vi "RydbergExpControl_2014.8.27_beta.vi"() -> ()   [LabVIEW 2013]
uses:
  AndorCamera/camera_controls.ctl
  <userlib>/atmcd32d.llb/AcquisitionMode_mode typedef.ctl
  <userlib>/atmcd32d.llb/TriggerMode_mode typedef.ctl
  6704/6704_static_voltages_control.ctl
  rydberg_state_machine_states.ctl
panel:
  out "Atom Closeup":dbl[][](graph)
  out "Atoms - BG":dbl[][](graph)
  out "error out":errorcluster
  out "error constant":errorcluster
  out "Array":dbl[](array[numeric])
  out "Background Image":i16[][](graph)
  out "Atom Image":i16[][](graph)
  in  "Tab Control":T1(tab)
  in  "Trigger Snap Mode":bool
  out "Camera Ready":bool
  in  "Scan Name":string
  in  "Raw_Data Folder":path
  out "Exp Running":bool
  in  "PB Instruction Time To Change":i32
  in  "Static Channel To Change":i32
  in  "Step Size":dbl min=1e-06
  in  "Final Value":dbl
  in  "Initial Value":dbl
  out "You Are Changing:":string
  in  "Shutdown Experiment":bool
  in  "Start Experiment":bool
  in  "Instructions":T2(array[cluster])=[{"Instruct Data"=0, "Op Code"=0, "Flags"=[TRUE, FALSE, FALSE, FALSE, FALSE, FALSE, FALSE, FALSE, FALSE, FALSE, FALSE, FALSE, FALSE, FALSE, FALSE, FALSE, FALSE, FALSE, FALSE, FALSE, FALSE, FALSE, FALSE, FALSE], "Comments"="", "Time (s)"=0.1}, {"Instruct Data"=0, "Op Code"=0, "Flags"=[FALSE, FALSE, FALSE, FALSE, FALSE, FALSE, FALSE, FALSE, FALSE, FALSE, FALSE, FALSE, FALSE, FALSE, FALSE, FALSE, FALSE, FALSE, FALSE, FALSE, FALSE, FALSE, FALSE, FALSE], "Comments"="", "Time (s)"=0.1}, {"Instruct Data"=0, "Op Code"=0, "Flags"=[TRUE, FALSE, FALSE, FALSE, FALSE, FALSE, FALSE, FALSE, FALSE, FALSE, FALSE, FALSE, FALSE, FALSE, FALSE, FALSE, FALSE, FALSE, FALSE, FALSE, FALSE, FALSE, FALSE, FALSE], "Comments"="", "Time (s)"=0.1}, {"Instruct Data"=0, "Op Code"=6, "Flags"=[FALSE, FALSE, FALSE, FALSE, FALSE, FALSE, FALSE, FALSE, FALSE, FALSE, FALSE, FALSE, FALSE, FALSE, FALSE, FALSE, FALSE, FALSE, FALSE, FALSE, FALSE, FALSE, FALSE, FALSE], "Comments"="", "Time (s)"=0.1}] {"Time (s)" format="%.3p"; "Op Code" items=["Continue", "Stop", "Loop", "End Loop", "JSR", "RTS", "Branch", "Long Delay", "Wait"]}
  in  "What To Change":enum16{"PulseBlaster", "Static Voltage"}(ring)=enum."Static Voltage"
  out "Scan Progress":dbl(slide) caption="Slide" scale=0.0..100.0
  out "Camera Information":T3 {"VS Speed (us)" format="%.2f"}
  in  "Acquisition Parameters":T4={"Acquisition Mode"=enum."Kinetics", "Trigger Mode"=enum."External", "Frame \nTransfer"=FALSE, "Exposure Time (s)"=0.0001, "Accumulation Cycle Time (s)"=0.0, "# Accumulations"=1, "# Kinetics"=2, "Kinetic Cycle Time (s)"=0.0, "Horizontal Bin Size"=1, "Vertical Bin Size"=1} {"Vertical Bin Size" min=1; "Horizontal Bin Size" min=1; "Kinetic Cycle Time (s)" format="%.2f"; "# Kinetics" min=1; "# Accumulations" min=1; "Accumulation Cycle Time (s)" format="%.2f"; "Exposure Time (s)" format="%.2e"}
  out "Calcualted Times":T7 {"Kinetic" format="%.4f"; "Accumulate" format="%.4f"; "Exposure" format="%.4f"}
  in  "Red MOT 87 Inputs":T8={"Active Device"="6733_Red_87", "Active Channels"=[TRUE, FALSE, FALSE, FALSE, FALSE, FALSE, FALSE, FALSE], "Waveform Parameters"=[[{"Functional Form"=enum."Polynomial", "Start Voltage"=0.0, "End Voltage"=0.0, "Time"=0.0, "Degree"=1, "Sample Rate"=0.0}, {"Functional Form"=enum."Exponential", "Start Voltage"=0.0, "End Voltage"=0.0, "Time"=0.0, "Degree"=1, "Sample Rate"=0.0}, {"Functional Form"=enum."Exponential", "Start Voltage"=0.0, "End Voltage"=0.0, "Time"=0.0, "Degree"=1, "Sample Rate"=0.0}, {"Functional Form"=enum."Exponential", "Start Voltage"=0.0, "End Voltage"=0.0, "Time"=0.0, "Degree"=1, "Sample Rate"=0.0}, {"Functional Form"=enum."Exponential", "Start Voltage"=0.0, "End Voltage"=0.0, "Time"=0.0, "Degree"=1, "Sample Rate"=0.0}, {"Functional Form"=enum."Exponential", "Start Voltage"=0.0, "End Voltage"=0.0, "Time"=0.0, "Degree"=1, "Sample Rate"=0.0}], [{"Functional Form"=enum."Exponential", "Start Voltage"=0.0, "End Voltage"=0.0, "Time"=0.0, "Degree"=1, "Sample Rate"=0.0}, {"Functional Form"=enum."Exponential", "Start Voltage"=0.0, "End Voltage"=0.0, "Time"=0.0, "Degree"=1, "Sample Rate"=0.0}, {"Functional Form"=enum."Exponential", "Start Voltage"=0.0, "End Voltage"=0.0, "Time"=0.0, "Degree"=1, "Sample Rate"=0.0}, {"Functional Form"=enum."Exponential", "Start Voltage"=0.0, "End Voltage"=0.0, "Time"=0.0, "Degree"=1, "Sample Rate"=0.0}, {"Functional Form"=enum."Exponential", "Start Voltage"=0.0, "End Voltage"=0.0, "Time"=0.0, "Degree"=1, "Sample Rate"=0.0}, {"Functional Form"=enum."Exponential", "Start Voltage"=0.0, "End Voltage"=0.0, "Time"=0.0, "Degree"=1, "Sample Rate"=0.0}], [{"Functional Form"=enum."Exponential", "Start Voltage"=0.0, "End Voltage"=0.0, "Time"=0.0, "Degree"=1, "Sample Rate"=0.0}, {"Functional Form"=enum."Exponential", "Start Voltage"=0.0, "End Voltage"=0.0, "Time"=0.0, "Degree"=1, "Sample Rate"=0.0}, {"Functional Form"=enum."Exponential", "Start Voltage"=0.0, "End Voltage"=0.0, "Time"=0.0, "Degree"=1, "Sample Rate"=0.0}, {"Functional Form"=enum."Exponential", "Start Voltage"=0.0, "End Voltage"=0.0, "Time"=0.0, "Degree"=1, "Sample Rate"=0.0}, {"Functional Form"=enum."Exponential", "Start Voltage"=0.0, "End Voltage"=0.0, "Time"=0.0, "Degree"=1, "Sample Rate"=0.0}, {"Functional Form"=enum."Exponential", "Start Voltage"=0.0, "End Voltage"=0.0, "Time"=0.0, "Degree"=1, "Sample Rate"=0.0}], [{"Functional Form"=enum."Exponential", "Start Voltage"=0.0, "End Voltage"=0.0, "Time"=0.0, "Degree"=1, "Sample Rate"=0.0}, {"Functional Form"=enum."Exponential", "Start Voltage"=0.0, "End Voltage"=0.0, "Time"=0.0, "Degree"=1, "Sample Rate"=0.0}, {"Functional Form"=enum."Exponential", "Start Voltage"=0.0, "End Voltage"=0.0, "Time"=0.0, "Degree"=1, "Sample Rate"=0.0}, {"Functional Form"=enum."Exponential", "Start Voltage"=0.0, "End Voltage"=0.0, "Time"=0.0, "Degree"=1, "Sample Rate"=0.0}, {"Functional Form"=enum."Exponential", "Start Voltage"=0.0, "End Voltage"=0.0, "Time"=0.0, "Degree"=1, "Sample Rate"=0.0}, {"Functional Form"=enum."Exponential", "Start Voltage"=0.0, "End Voltage"=0.0, "Time"=0.0, "Degree"=1, "Sample Rate"=0.0}], [{"Functional Form"=enum."Exponential", "Start Voltage"=0.0, "End Voltage"=0.0, "Time"=0.0, "Degree"=1, "Sample Rate"=0.0}, {"Functional Form"=enum."Exponential", "Start Voltage"=0.0, "End Voltage"=0.0, "Time"=0.0, "Degree"=1, "Sample Rate"=0.0}, {"Functional Form"=enum."Exponential", "Start Voltage"=0.0, "End Voltage"=0.0, "Time"=0.0, "Degree"=1, "Sample Rate"=0.0}, {"Functional Form"=enum."Exponential", "Start Voltage"=0.0, "End Voltage"=0.0, "Time"=0.0, "Degree"=1, "Sample Rate"=0.0}, {"Functional Form"=enum."Exponential", "Start Voltage"=0.0, "End Voltage"=0.0, "Time"=0.0, "Degree"=1, "Sample Rate"=0.0}, {"Functional Form"=enum."Exponential", "Start Voltage"=0.0, "End Voltage"=0.0, "Time"=0.0, "Degree"=1, "Sample Rate"=0.0}], [{"Functional Form"=enum."Exponential", "Start Voltage"=0.0, "End Voltage"=0.0, "Time"=0.0, "Degree"=1, "Sample Rate"=0.0}, {"Functional Form"=enum."Exponential", "Start Voltage"=0.0, "End Voltage"=0.0, "Time"=0.0, "Degree"=1, "Sample Rate"=0.0}, {"Functional Form"=enum."Exponential", "Start Voltage"=0.0, "End Voltage"=0.0, "Time"=0.0, "Degree"=1, "Sample Rate"=0.0}, {"Functional Form"=enum."Exponential", "Start Voltage"=0.0, "End Voltage"=0.0, "Time"=0.0, "Degree"=1, "Sample Rate"=0.0}, {"Functional Form"=enum."Exponential", "Start Voltage"=0.0, "End Voltage"=0.0, "Time"=0.0, "Degree"=1, "Sample Rate"=0.0}, {"Functional Form"=enum."Exponential", "Start Voltage"=0.0, "End Voltage"=0.0, "Time"=0.0, "Degree"=1, "Sample Rate"=0.0}], [{"Functional Form"=enum."Exponential", "Start Voltage"=0.0, "End Voltage"=0.0, "Time"=0.0, "Degree"=1, "Sample Rate"=0.0}, {"Functional Form"=enum."Exponential", "Start Voltage"=0.0, "End Voltage"=0.0, "Time"=0.0, "Degree"=1, "Sample Rate"=0.0}, {"Functional Form"=enum."Exponential", "Start Voltage"=0.0, "End Voltage"=0.0, "Time"=0.0, "Degree"=1, "Sample Rate"=0.0}, {"Functional Form"=enum."Exponential", "Start Voltage"=0.0, "End Voltage"=0.0, "Time"=0.0, "Degree"=1, "Sample Rate"=0.0}, {"Functional Form"=enum."Exponential", "Start Voltage"=0.0, "End Voltage"=0.0, "Time"=0.0, "Degree"=1, "Sample Rate"=0.0}, {"Functional Form"=enum."Exponential", "Start Voltage"=0.0, "End Voltage"=0.0, "Time"=0.0, "Degree"=1, "Sample Rate"=0.0}], [{"Functional Form"=enum."Exponential", "Start Voltage"=0.0, "End Voltage"=0.0, "Time"=0.0, "Degree"=1, "Sample Rate"=0.0}, {"Functional Form"=enum."Exponential", "Start Voltage"=0.0, "End Voltage"=0.0, "Time"=0.0, "Degree"=1, "Sample Rate"=0.0}, {"Functional Form"=enum."Exponential", "Start Voltage"=0.0, "End Voltage"=0.0, "Time"=0.0, "Degree"=1, "Sample Rate"=0.0}, {"Functional Form"=enum."Exponential", "Start Voltage"=0.0, "End Voltage"=0.0, "Time"=0.0, "Degree"=1, "Sample Rate"=0.0}, {"Functional Form"=enum."Exponential", "Start Voltage"=0.0, "End Voltage"=0.0, "Time"=0.0, "Degree"=1, "Sample Rate"=0.0}, {"Functional Form"=enum."Exponential", "Start Voltage"=0.0, "End Voltage"=0.0, "Time"=0.0, "Degree"=1, "Sample Rate"=1.0}]], "Active Phases"=[TRUE, FALSE, FALSE, FALSE, FALSE, FALSE], "Phase Times"=[0.001], "Trigger Channel"="/6733_Red_87/PFI0"} {"Phase Times" format="%.0p"; "Waveform Parameters"."Degree" min=1}
  in  "6704 Static Voltage Settings":T9={"Device Name"="6704_Static", "Voltages"=[5.0, 0.0, 0.0, 0.0, 0.0, 0.0, 0.0, 0.0, 0.0, 0.0, 0.0, 0.0, 0.0, 0.0, 0.0, 0.0]}
  out "Andor Initialization Error Codes":T10
  out "Acq. Error Codes":T11
  out "Tree":string(tree)
  # "(1) 461 MOT beams"
  # "(2) Imaging AOM 1"
  # "(3) Imaging AOM 2"
  # "(4) Camera"
  # "(5) Zeeman shutter"
  # "(6) Repumper shutter"
  # "(7) 461 MOT coils"
  # "(8) 689 MOT coils"
  # "(9) 87 Sr Red MOT Trig"
  # "(10) ??? Shutter"
  # "(11) Red AOM"
  # "(12) Sat Abs Current Switch"
  # "(13) Zeeman MOSFET"
  # "1"
  # "2"
  # "3"
  # "4"
  # "5"
  # "6"
  # "7"
  # "8"
  # "9"
  # "10"
  # "11"
  # "12"
  # "13"
  # "14"
  # "15"
  # "16"
  # "17"
  # "18"
  # "19"
  # "20"
  # "21"
  # "22"
  # "23"
  # "24"
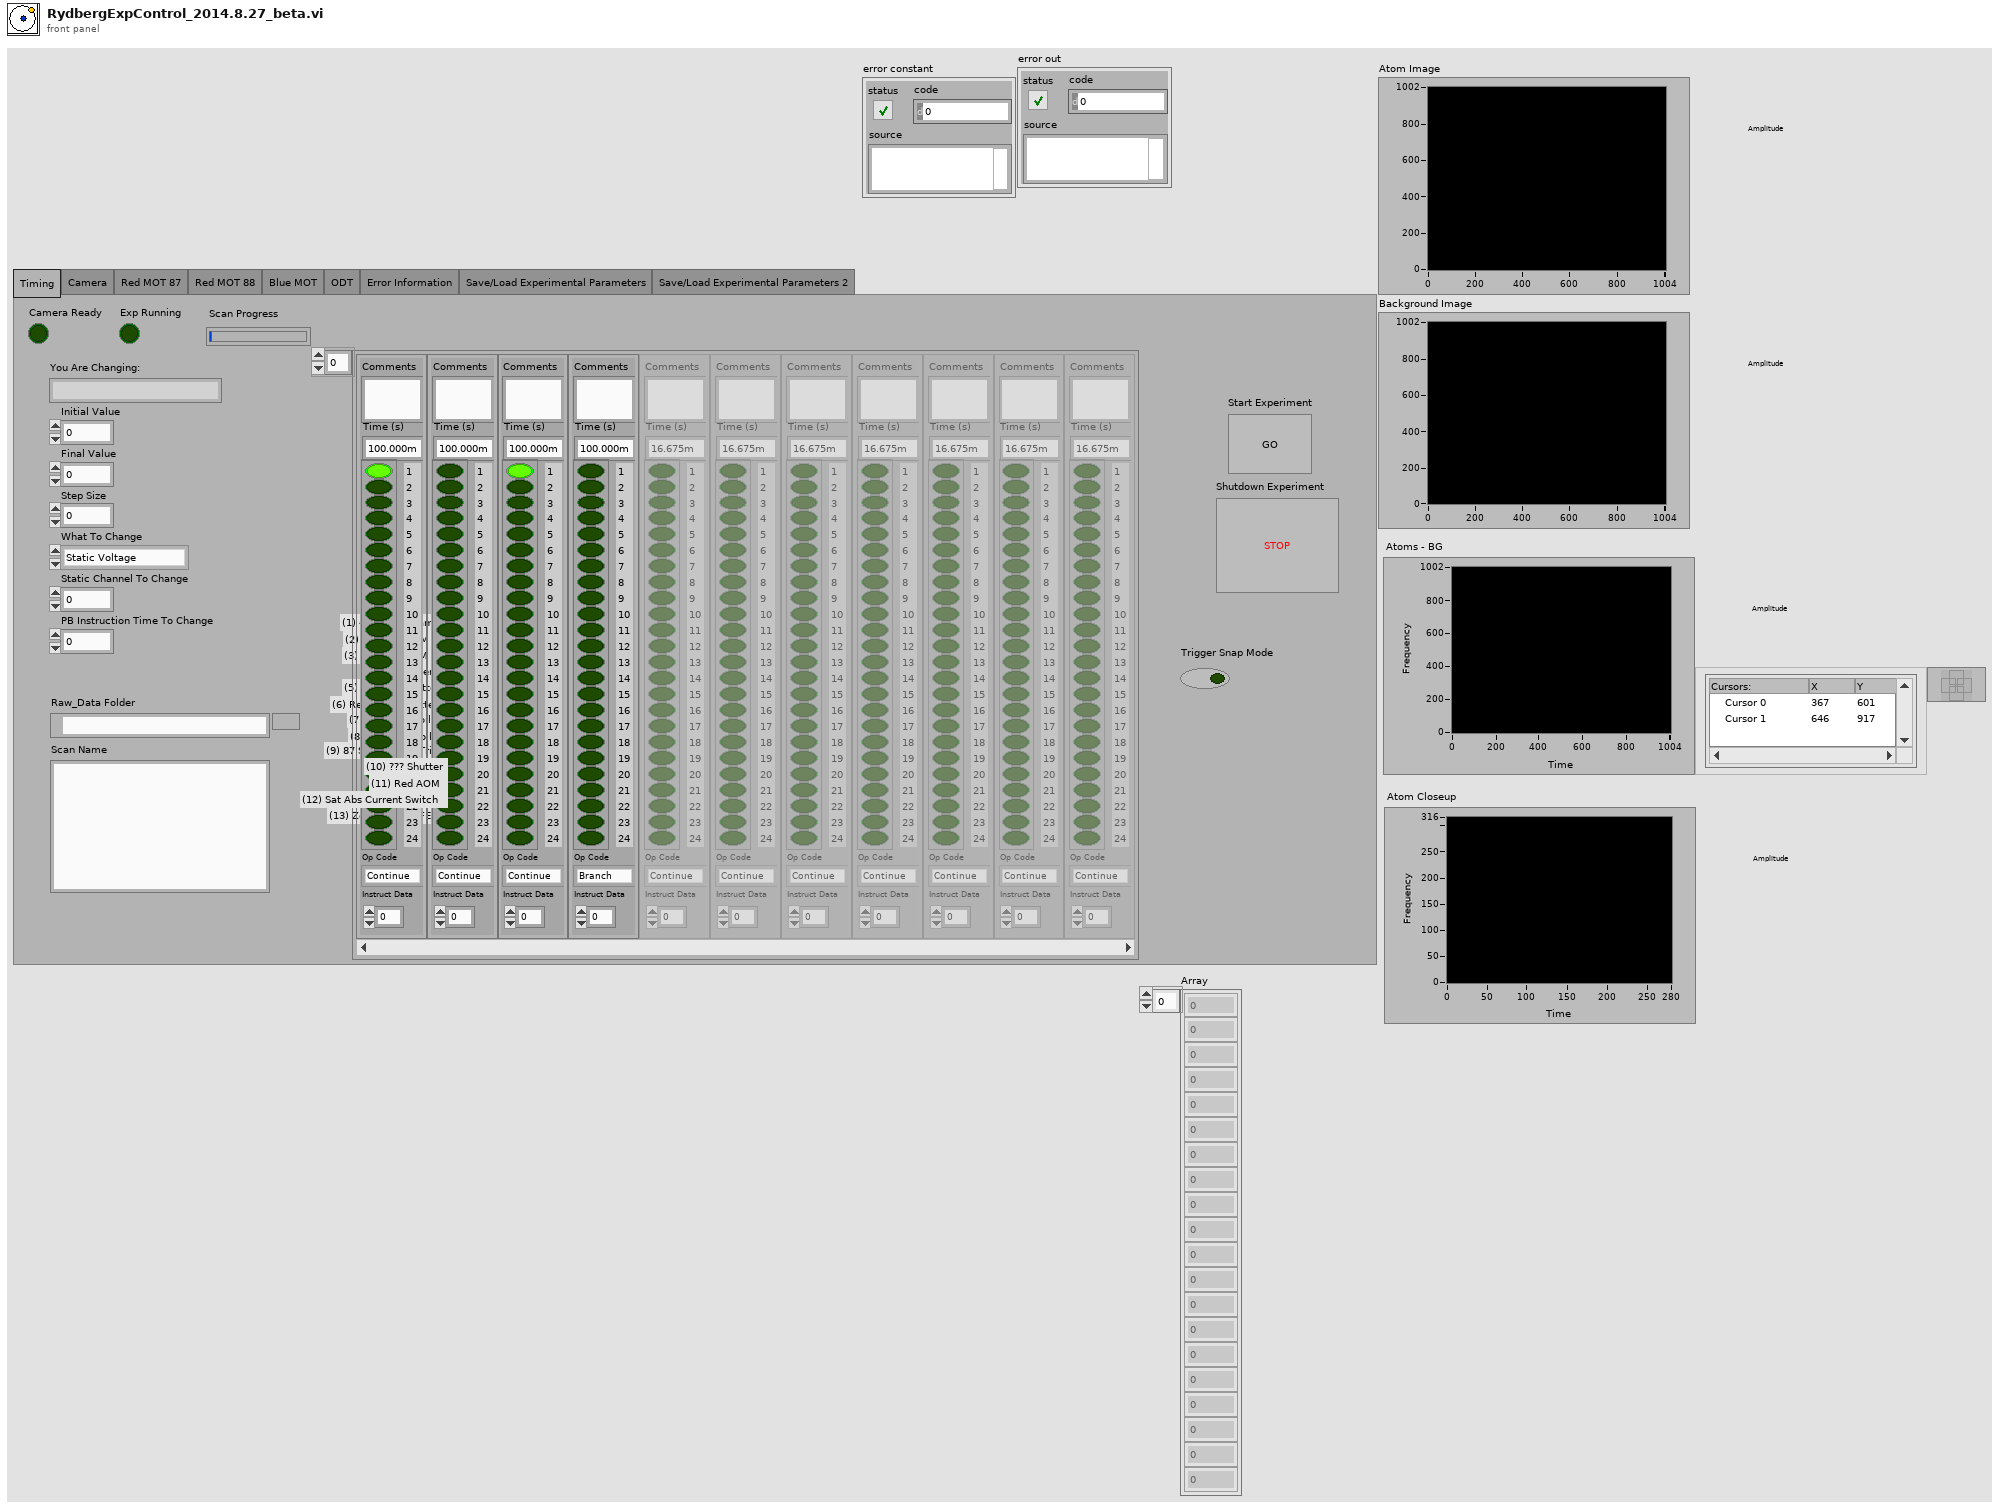
[diagram p1: front panel]
types:
  T1 = enum32{"Timing", "Camera", "Red MOT 87", "Red MOT 88", "Blue MOT", "ODT", "Error Information", "Save/Load Experimental Parameters", "Save/Load Experimental Parameters 2"}
  T2 = cluster{"Instruct Data":i32, "Op Code":i32, "Flags":bool[], "Comments":string, "Time (s)":dbl}[]
  T3 = cluster{"xpixels":i32, "ypixels":i32, "# VS Speeds":i32, "VS Speed (us)":sgl, "Temperature Stable":bool, "Temperature (C)":i32}
  T4 = typedef "camera_controls.ctl" = cluster{"Acquisition Mode":T5, "Trigger Mode":T6, "Frame \nTransfer":bool, "Exposure Time (s)":sgl, "Accumulation Cycle Time (s)":sgl, "# Accumulations":i32, "# Kinetics":i32, "Kinetic Cycle Time (s)":sgl, "Horizontal Bin Size":i32, "Vertical Bin Size":i32}
  T5 = typedef "AcquisitionMode_mode typedef.ctl" = enum16{"Reserved (0)", "Single Scan", "Accumulate", "Kinetics", "Fast Kinetics", "Run Till Abort", "Reserved (6)", "Reserved (7)", "Reserved (8)", "Time Delayed Integration"}
  T6 = typedef "TriggerMode_mode typedef.ctl" = enum16{"Internal", "External", "N/A (2)", "N/A (3)", "N/A (4)", "N/A (5)", "External Start", "External Exposure (Bulb)", "N/A (8)", "External FVB EM", "Software", "N/A (11)", "External Charge Shifting"}
  T7 = cluster{"Exposure":sgl, "Accumulate":sgl, "Kinetic":sgl}
  T8 = cluster{"Active Device":string, "Active Channels":bool[], "Waveform Parameters":cluster{"Functional Form":enum16{"Polynomial", "Exponential"}, "Start Voltage":dbl, "End Voltage":dbl, "Time":dbl, "Degree":i8, "Sample Rate":dbl}[][], "Active Phases":bool[], "Phase Times":dbl[], "Trigger Channel":tag}
  T9 = typedef "6704_static_voltages_control.ctl" = cluster{"Device Name":string, "Voltages":dbl[]}
  T10 = cluster{"Initalize Error Code":u32, "GetDetector Error Code":u32, "Get#VSSpeeds Error Code":u32, "Set VS Speed Error":u32, "CoolerOn Error Code":u32, "GetTemperature Error Code":u32, "Shutdown Error Code":u32}
  T11 = cluster{"Set Acq. Mode Error":u32, "Set Trigger Mode Error":u32, "Set FT Error Code":u32, "Set Exposure Time Error Code":u32, "Set Accum Time Error":u32, "Set # Accum Error":u32, "Set # Kinetics Error":u32, "SetKinCycleTime Error":u32}
  T12 = typedef "rydberg_state_machine_states.ctl" = enum16{"Initialize", "Idle", "Trigger Snap Mode", "Scan Mode", "Load Experiment", "Shutdown"}
  T13 = cluster{"6704 Static Voltage Settings":T9, "Instructions":cluster{"Instruct Data":i32, "Op Code":i32, "Flags":bool[], "Comments":string, "Time (s)":dbl}[], "Red MOT 87 Inputs":cluster{"Active Device":string, "Active Channels":bool[], "Waveform Parameters":cluster{"Functional Form":enum16{"Polynomial", "Exponential"}, "Start Voltage":dbl, "End Voltage":dbl, "Time":dbl, "Degree":i8, "Sample Rate":dbl}[][], "Active Phases":bool[], "Phase Times":dbl[], "Trigger Channel":tag}}
  T14 = typedef "LVCursorListTypeDef.ctl" = cluster{"Name":string, "Color":u32, "Style":u8, "Point Style":u8, "Name Visible":bool, "Allow Drag":bool, "Cursor Mode":u32, "Plot":i32, "Index":i32, "Position":cluster{"X":dbl, "Y":dbl}, "X Scale":u32, "Y Scale":u32, "Watch Plots":i32[], "Watch All Plots":bool, "Plot Area":i32, "Label Offset":cluster{"X":dbl, "Y":dbl}}[]
  T15 = cluster{"Instruct Data":i32, "Op Code":i32, "Flags":bool[], "Comments":string, "Time (s)":dbl}
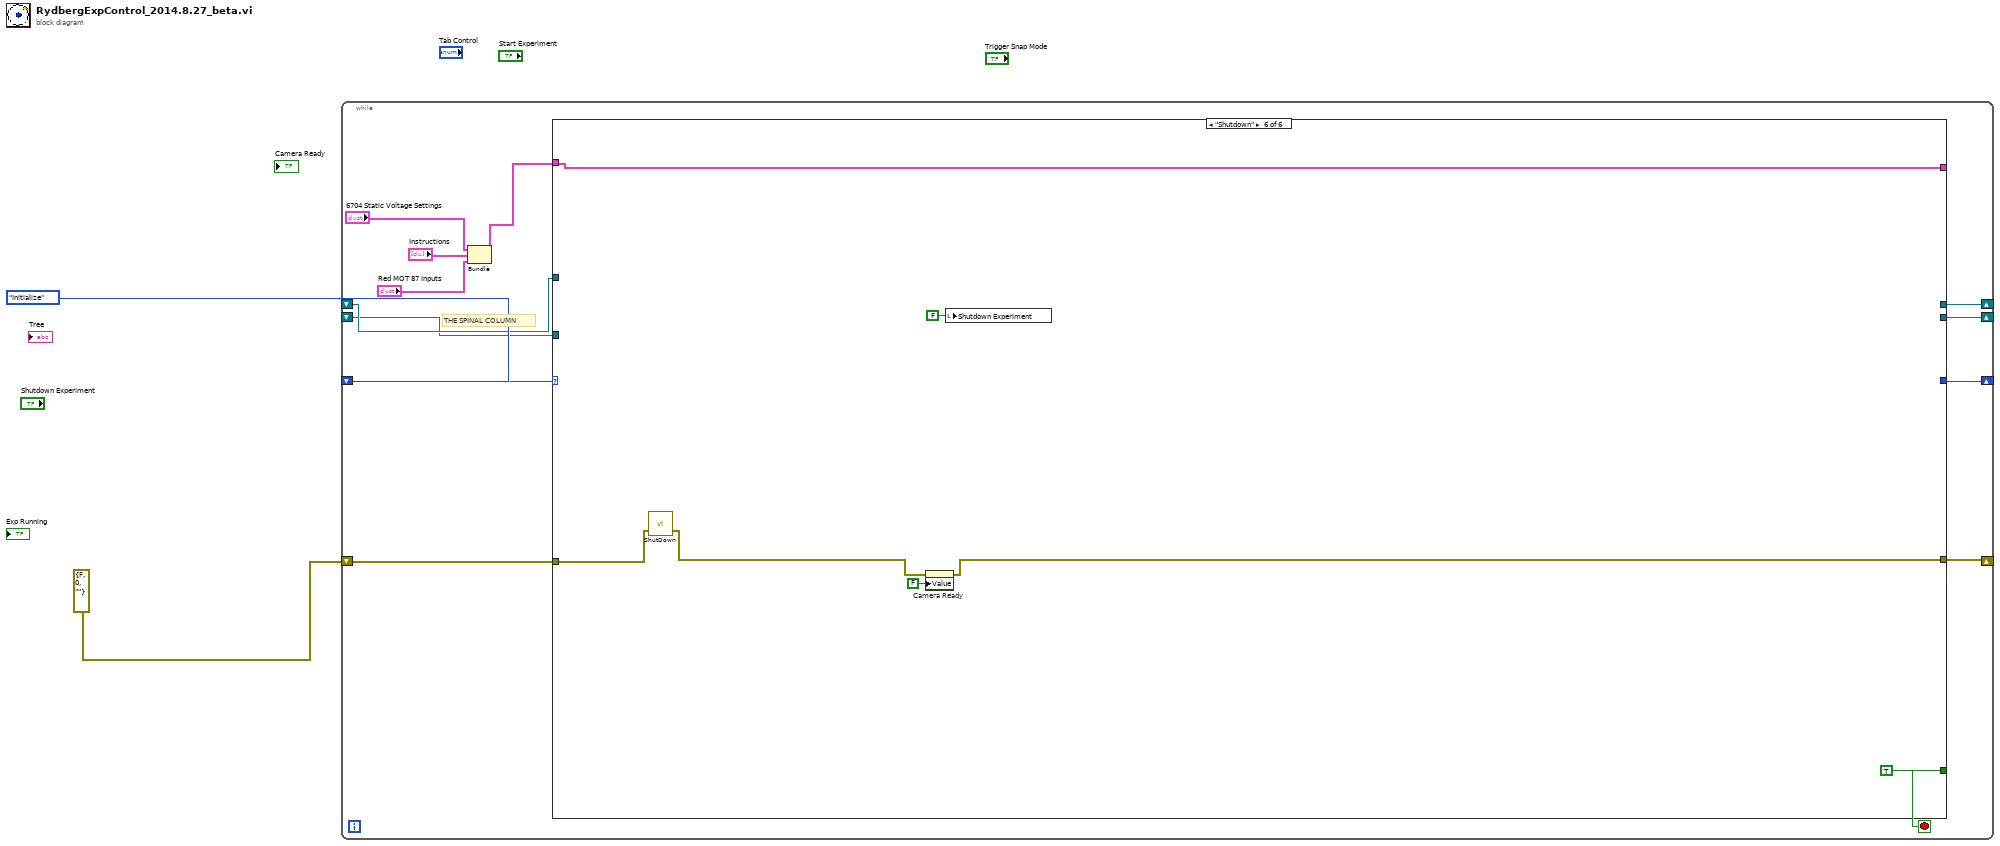
[diagram p0: block diagram]
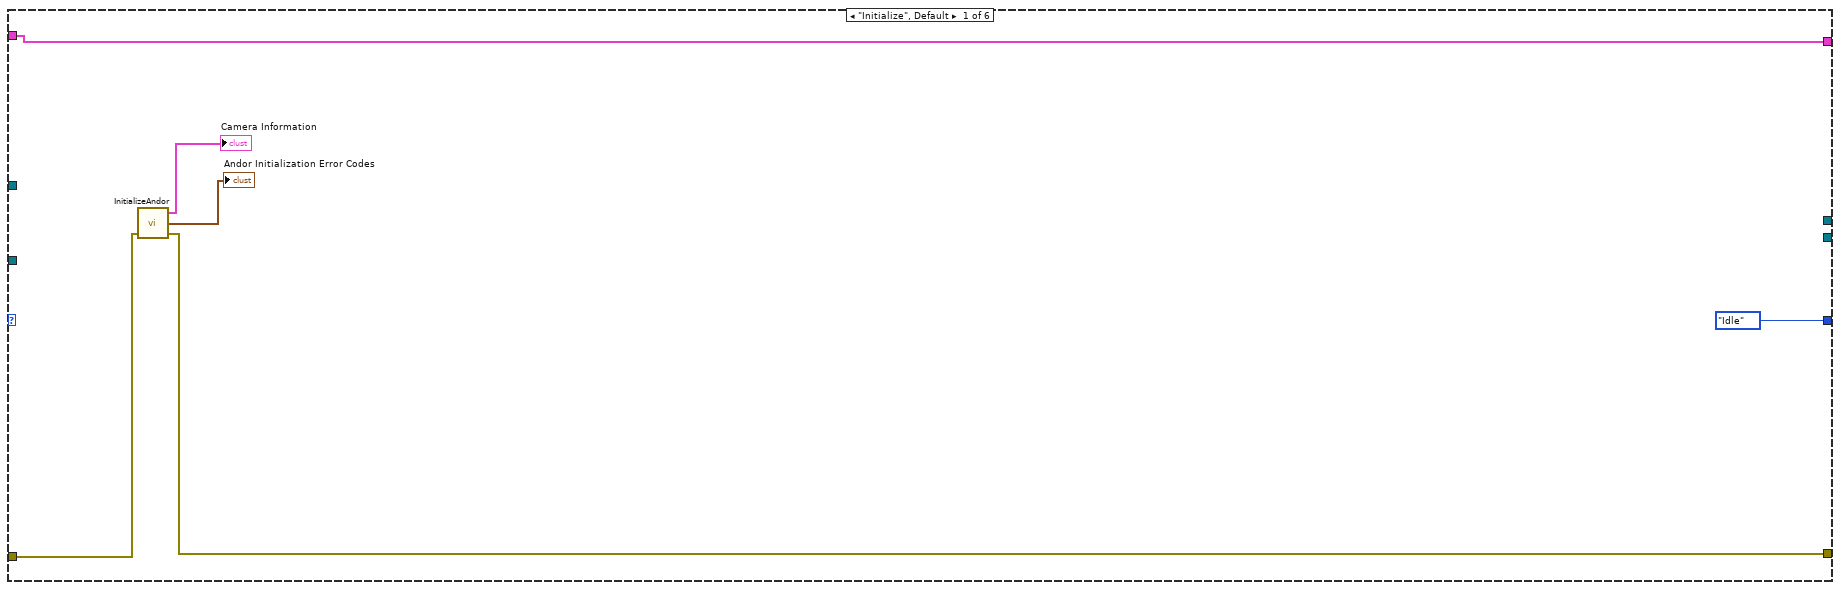
[diagram p2: hidden frame]
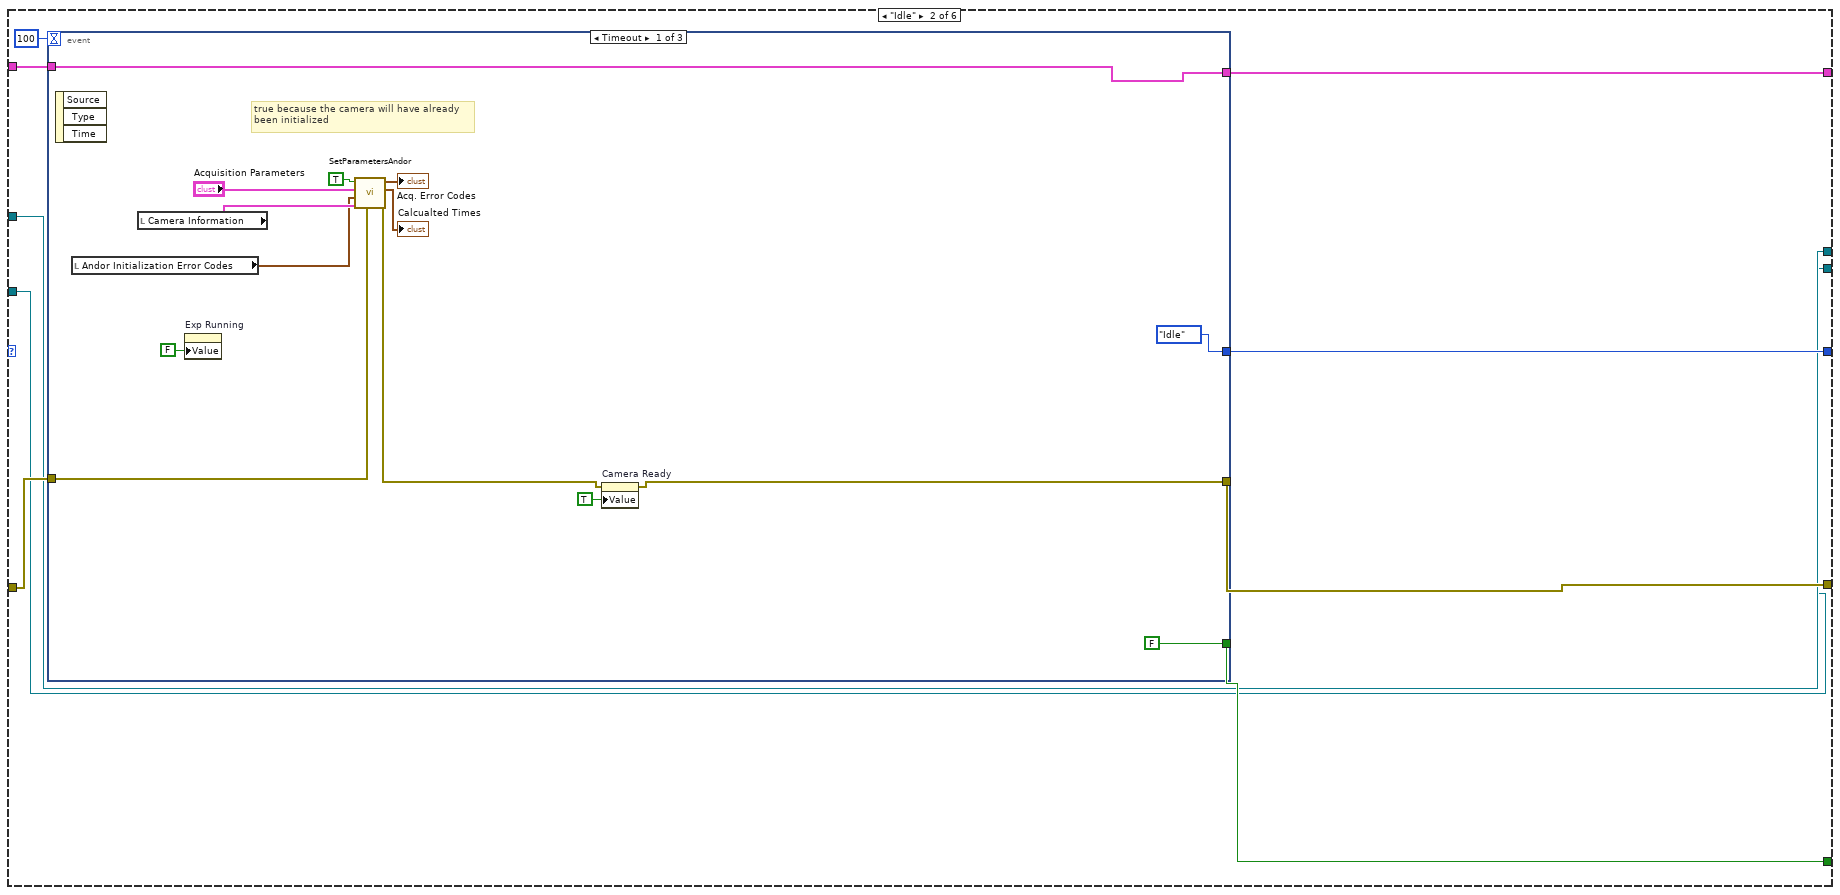
[diagram p3: hidden frame]
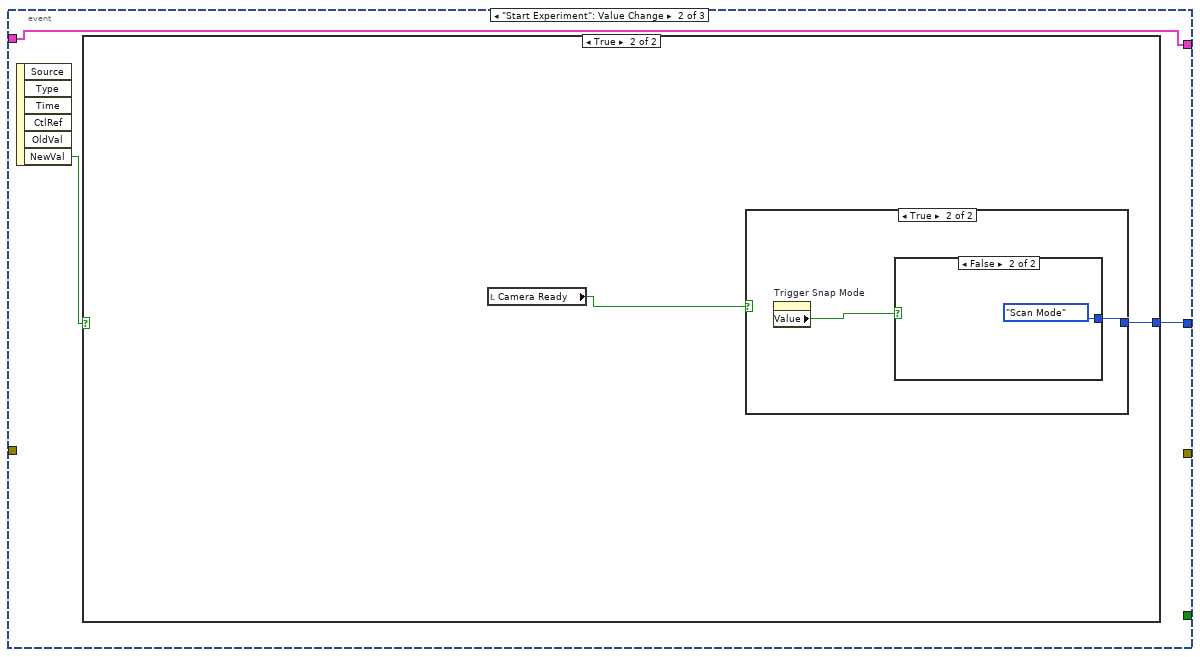
[diagram p4: hidden frame]
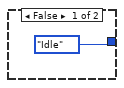
[diagram p5: hidden frame]
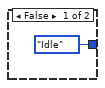
[diagram p6: hidden frame]
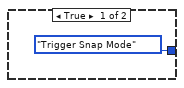
[diagram p7: hidden frame]
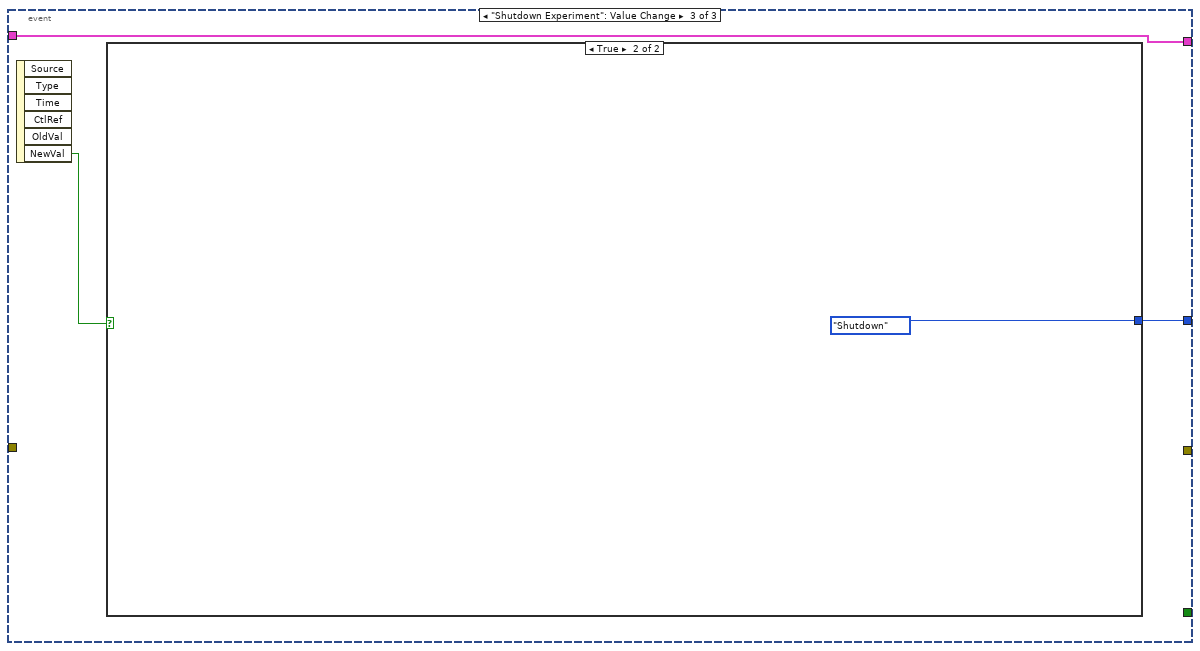
[diagram p8: hidden frame]
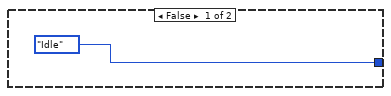
[diagram p9: hidden frame]
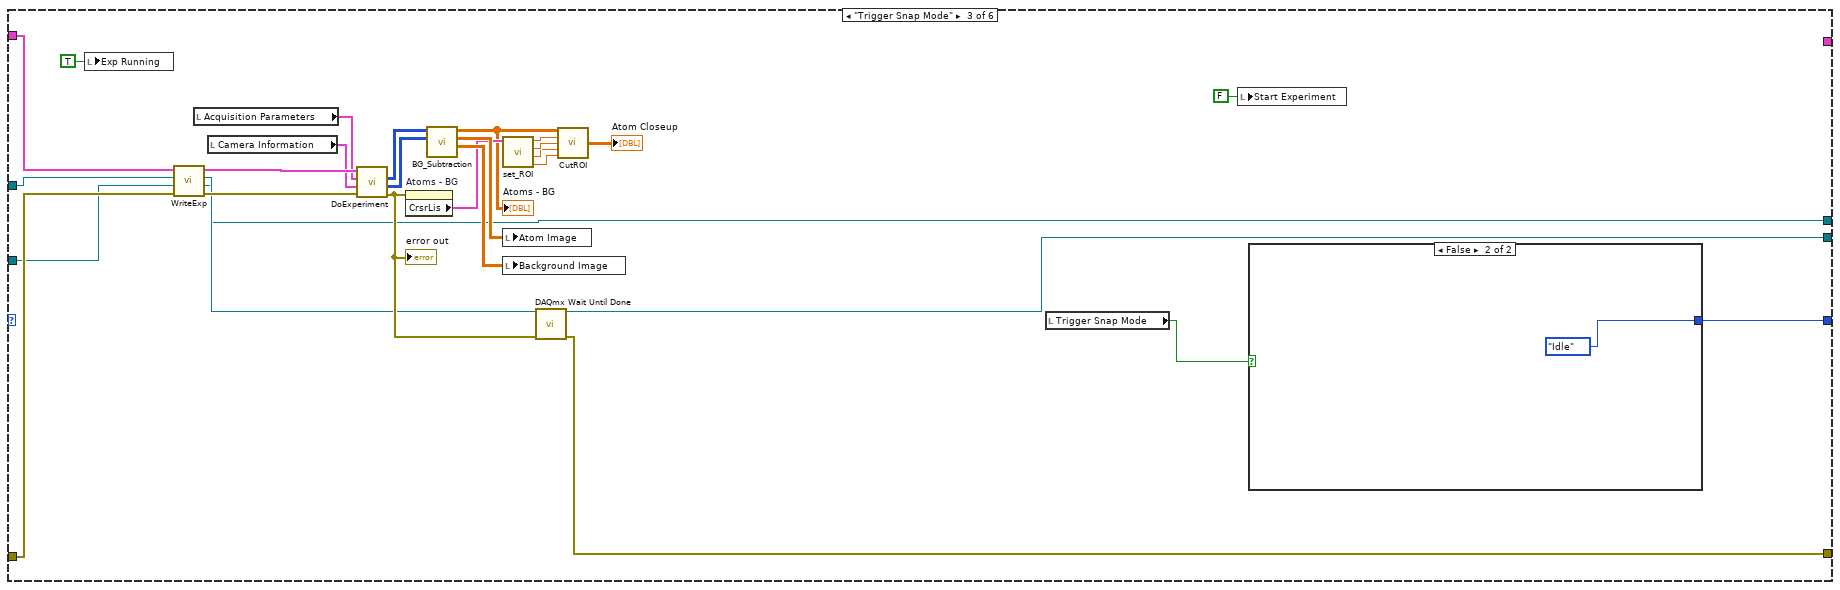
[diagram p10: hidden frame]
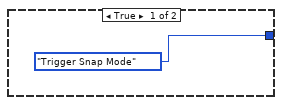
[diagram p11: hidden frame]
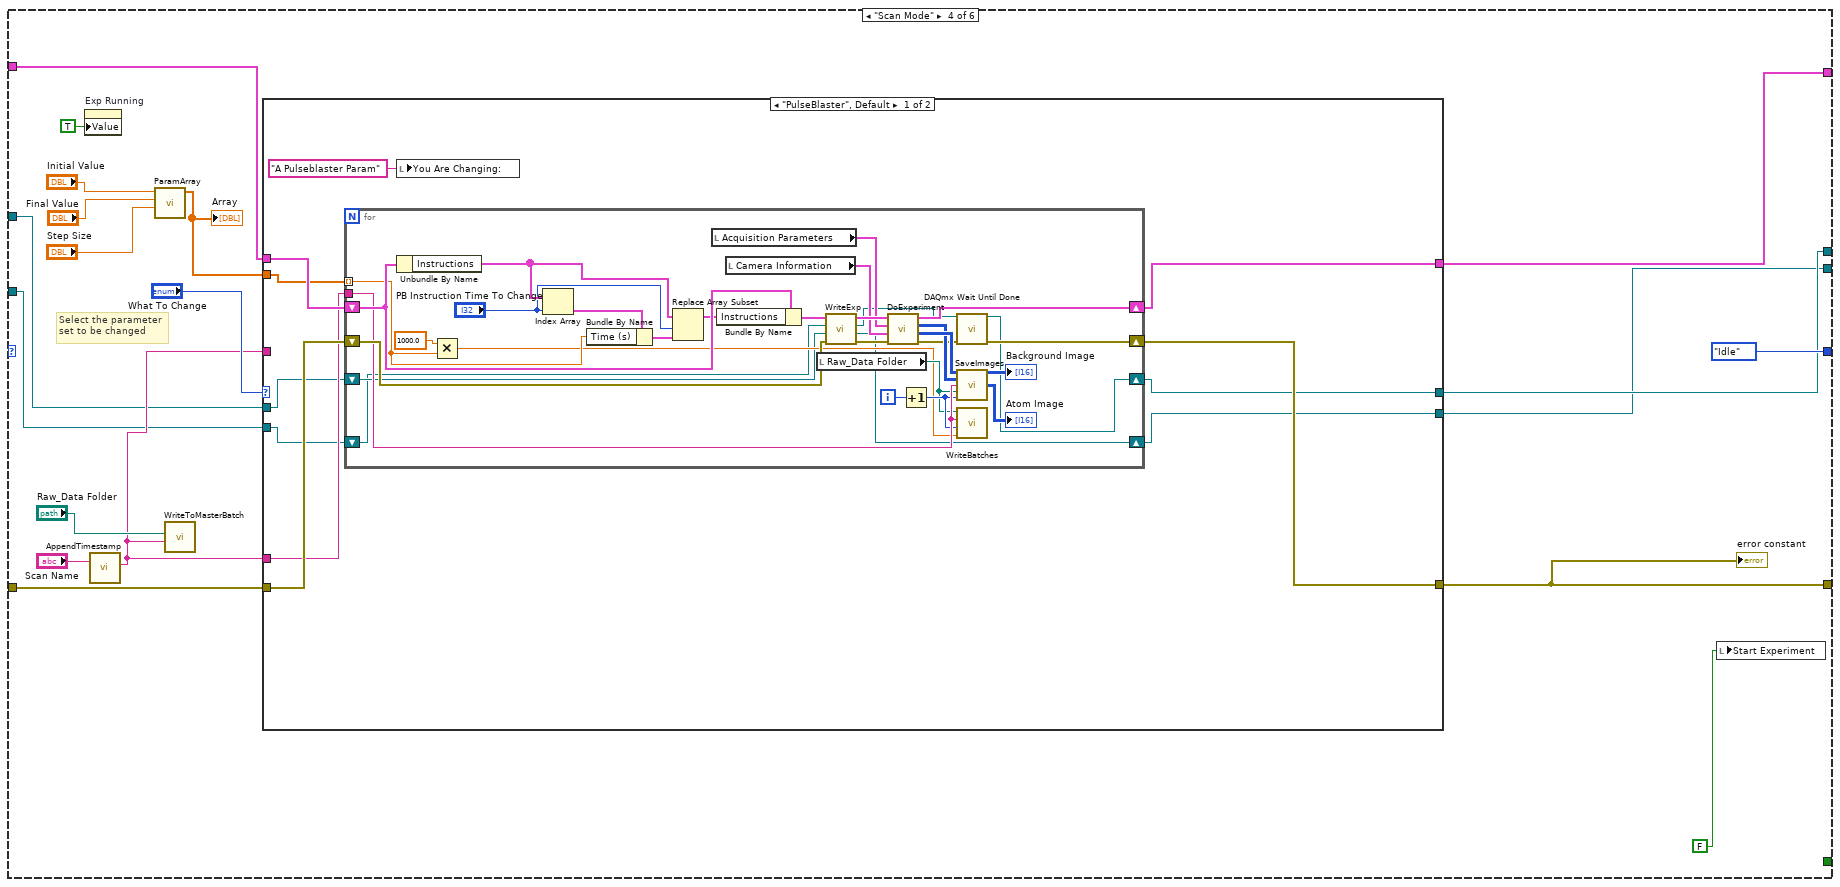
[diagram p12: hidden frame]
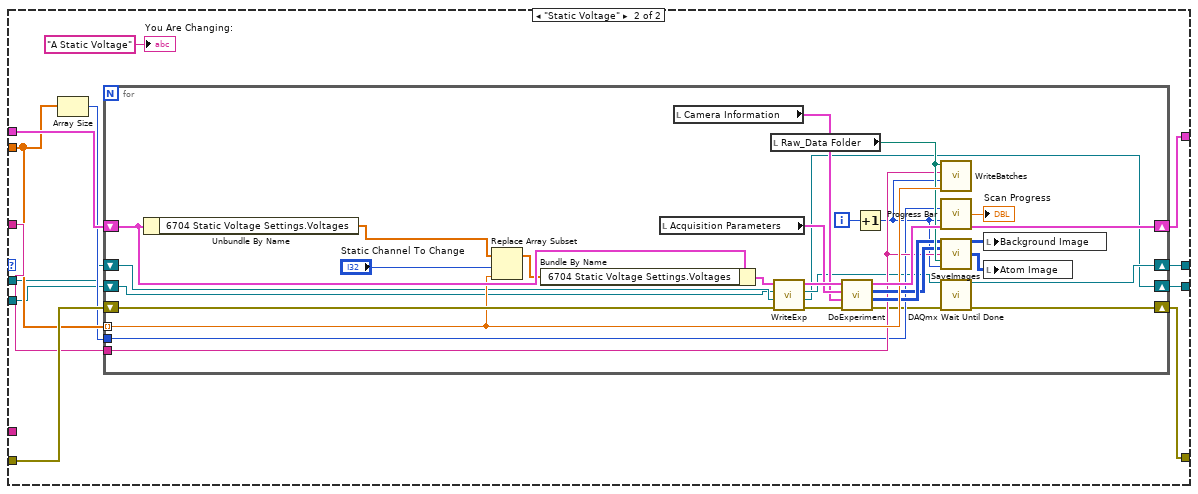
[diagram p13: hidden frame]
diagram:
  n1 = while {
    shift-right: [w12] -> _
    shift-left: rydberg_state_machine_states."Initialize" -> [w15]
    shift-right: [w13] -> _
    shift-left: errorcluster {"status"=FALSE, "code"=0, "source"=""} ("error constant") -> [w14]
    shift-right: [w6] -> _
    shift-left: _ -> [w5]
    shift-right: [w4] -> _
    shift-left: _ -> [w3]
    stop <- w11 stop-if-true
    # "THE SPINAL COLUMN"
    n2 = Bundle("6704 Static Voltage Settings"="6704 Static Voltage Settings", "Instructions"="Instructions", "Red MOT 87 Inputs"="Red MOT 87 Inputs") -> (w7:T13)  [unwired: 1 in]
    n3 = case shown="\"Shutdown\"" w15 {
      tunnel: w14 -> [w21 w30 w88 w101 _ w200]
      tunnel: [w18 w26 w61 w100 _ w195] -> w13
      tunnel: [rydberg_state_machine_states."Idle" w28 w71 rydberg_state_machine_states."Idle" _ _] -> w12
      tunnel: [_ w27 _ _ _ TRUE] -> w11
      tunnel: [w16 w25 _ w103 w193 w197] -> _
      tunnel: w7 -> [w16 w24 w87 w104 w193 w197]
      tunnel: [_ w23 w65 w92 _ _] -> w6
      tunnel: w5 -> [_ w23 w64 w94 _ _]
      tunnel: [_ w22 w63 w91 _ _] -> w4
      tunnel: w3 -> [_ w22 w62 w93 _ _]
      frame "Initialize", Default {
        n4 = call "InitializeAndor.vi"("Error In"=w21) -> ("error out"=w18:errorcluster, "Andor Initialization Error Codes"=→"Andor Initialization Error Codes":T10, "Camera Information"=→"Camera Information":T3)  [unwired: 2 in]
      }
      frame "Idle" {
        n5 = event shown="[0] Timeout" {
          selector: _ -> [_ _ _]
          dyn-events: _ -> [_ _ _]
          timeout: 100 -> [_ _ _]
          tunnel: w30 -> [w38 _ _]
          tunnel: [rydberg_state_machine_states."Idle" w46 w57] -> w28
          tunnel: [FALSE _ _] -> w27
          tunnel: [w32 _ _] -> w26
          tunnel: [w35 w45 w56] -> w25
          tunnel: w24 -> [w35 w45 w56]
          event Timeout {
            # "true because the camera will have already\nbeen initialized"
            n6 = event-data() -> ()  [unwired: 1 in, 3 out]
            n7 = local read "Andor Initialization Error Codes"() -> (w37:T10)
            n8 = local read "Camera Information"() -> (w40:T3)
            n9 = property on="Exp Running" class="Bool (strict)"("Value"=FALSE ("Exp Running")) -> ()  [unwired: 2 in, 2 out]
            n10 = call "SetParametersAndor.vi"("Error In"=w38, "Camera Information"=w40, "Andor Initialization Error Codes"=w37, "Acquisition Parameters"="Acquisition Parameters", "Pre Initialized?"=TRUE) -> ("error out"=w33:errorcluster, "Calcualted Times"=→"Calcualted Times":T7, "Acq. Error Codes"=→"Acq. Error Codes":T11)  [unwired: 4 in]
            n11 = property on="Camera Ready" class="Bool (strict)"(error in=w33, "Value"=TRUE ("Camera Ready")) -> (error out=w32:errorcluster)  [unwired: 1 in, 1 out]
          }
          event "Start Experiment": Value Change {
            n12 = event-data() -> ("NewVal"=w47:bool)  [unwired: 1 in, 5 out]
            n13 = case shown="True" w47 {
              tunnel: [rydberg_state_machine_states."Idle" w50] -> w46
              frame False {
              }
              frame True {
                n14 = local read "Camera Ready"() -> (w49:bool)
                n15 = case shown="True" w49 {
                  tunnel: [rydberg_state_machine_states."Idle" w53] -> w50
                  frame False {
                  }
                  frame True {
                    n16 = property on="Trigger Snap Mode" class="Bool (strict)"() -> ("Value"=w52:bool)  [unwired: 2 in, 2 out]
                    n17 = case shown="False" w52 {
                      tunnel: [rydberg_state_machine_states."Trigger Snap Mode" rydberg_state_machine_states."Scan Mode"] -> w53
                      frame True {
                      }
                      frame False {
                      }
                    }
                  }
                }
              }
            }
          }
          event "Shutdown Experiment": Value Change {
            n18 = event-data() -> ("NewVal"=w58:bool)  [unwired: 1 in, 5 out]
            n19 = case shown="True" w58 {
              tunnel: [rydberg_state_machine_states."Idle" rydberg_state_machine_states."Shutdown"] -> w57
              frame False {
              }
              frame True {
              }
            }
          }
        }
      }
      frame "Trigger Snap Mode" {
        n20 = local write "Exp Running"(TRUE ("Exp Running")) -> ()
        n21 = call "WriteExp.vi"("error in (no error)"=w88, "Control Task In"=w62, "Waveform Task In"=w64, "Experimental Control Cluster In"=w87) -> ("error out"=w68:errorcluster, "waveform task out"=w65:refnum<k21>, "counter task out"=w66:refnum<k21>, "Experimental Control Cluster Out"=w86:T13)  [unwired: 4 in]
        n22 = local read "Acquisition Parameters"() -> (w85:T4)
        n23 = local read "Camera Information"() -> (w84:T3)
        n24 = call "DoExperiment.vi"("Error In"=w68, "Camera Information 2"=w84, "Acquisition Parameters"=w85, "output cluster"=w86) -> ("error out"=w67:errorcluster, "Background Image"=w82:i32[][], "Atom Image"=w83:i32[][])  [unwired: 4 in, 1 out]
        "error out" <- w67
        n25 = property on="Atoms - BG" class="IntGraph (strict)"(error in=w67) -> ("CrsrLis"=w79:T14)  [unwired: 1 in, 2 out]
        n26 = call "BG_Subtraction.vi"("Background Image"=w82, "Atom Image"=w83) -> ("Background Image Out"=w80:dbl[][], "Atom Image Out"=w81:dbl[][], "Atoms - BG"=w77:dbl[][])  [unwired: 7 in]
        "Atoms - BG" <- w77
        n27 = call "set_ROI.vi"("Cursor List"=w79) -> ("Row End"=w73:dbl, "RowStart"=w74:dbl, "ColEnd"=w75:dbl, "ColStart"=w76:dbl)  [unwired: 7 in]
        n28 = local write "Atom Image"(w81) -> ()
        n29 = local write "Background Image"(w80) -> ()
        n30 = call <vilib>:"DAQmx Wait Until Done.vi"("task/channels in"=w66, "error in"=w67) -> ("task out"=w63:refnum<k21>, "error out"=w61:errorcluster)  [unwired: 12 in]
        n31 = call "CutROI.vi"("Full Image In"=w77, "Col Start"=w76, "Col End"=w75, "Row Start"=w74, "Row End"=w73) -> ("Cut Image Out"=→"Atom Closeup":dbl[][])  [unwired: 10 in]
        n32 = local read "Trigger Snap Mode"() -> (w72:bool)
        n33 = local write "Start Experiment"(FALSE ("Start Experiment")) -> ()
        n34 = case shown="False" w72 {
          tunnel: [rydberg_state_machine_states."Trigger Snap Mode" rydberg_state_machine_states."Idle"] -> w71
          frame True {
          }
          frame False {
          }
        }
      }
      frame "Scan Mode" {
        # "Select the parameter\nset to be changed"
        n35 = property on="Exp Running" class="Bool (strict)"("Value"=TRUE ("Exp Running")) -> ()  [unwired: 2 in, 2 out]
        n36 = call "AppendTimestamp.vi"("String"="Scan Name") -> ("String 2"=w95:string)  [unwired: 10 in]
        n37 = call "ParamArray.vi"("Step Size"="Step Size", "Final Value"="Final Value", "Initial Value"="Initial Value") -> ("Array"=w102:dbl[])  [unwired: 8 in]
        "Array" <- w102
        n38 = call "WriteToMasterBatch.vi"("Scan name"=w95, "Raw_Data Folder"="Raw_Data Folder") -> ()  [unwired: 10 in]
        n39 = case shown="\"PulseBlaster\", Default" "What To Change" {
          tunnel: w104 -> [w119 w162]
          tunnel: [w117 w161] -> w103
          tunnel: w102 -> [w118 w157]
          tunnel: w101 -> [w116 w159]
          tunnel: [w115 w160] -> w100
          tunnel: w95 -> [_ w158]
          tunnel: w95 -> [w114 _]
          tunnel: w94 -> [w113 w155]
          tunnel: w93 -> [w112 w154]
          tunnel: [w111 w153] -> w92
          tunnel: [w110 w152] -> w91
          frame "PulseBlaster", Default {
            n40 = for {
              tunnel: w118 -> [w130] mode=indexing
              shift-right: [w141] -> w117
              shift-left: w119 -> [w147]
              shift-right: [w123] -> w115
              shift-left: w116 -> [w144]
              tunnel: w114 -> [w135]
              shift-right: [w122] -> w111
              shift-left: w113 -> [w127]
              shift-right: [w121] -> w110
              shift-left: w112 -> [w126]
              i -> [w138]
              n41 = Unbundle By Name(w147) -> ("Instructions"=w149:T2)
              n42 = Multiply(x=1000.0, y=w130) -> (x*y=w128:dbl)
              n43 = Index Array(array=w149, index="PB Instruction Time To Change") -> (element=w151:T15)
              n44 = Bundle By Name(cluster=w151, "Time (s)"=w130) -> (w150:T15)
              n45 = Replace Array Subset(array=w149, new element=w150, index="PB Instruction Time To Change") -> (w146:T2)
              n46 = local read "Acquisition Parameters"() -> (w140:T4)
              n47 = Bundle By Name(cluster=w147, "Instructions"=w146) -> (w145:T13)
              n48 = local read "Camera Information"() -> (w139:T3)
              n49 = local read "Raw_Data Folder"() -> (w133:path)
              n50 = call "WriteExp.vi"("error in (no error)"=w144, "Control Task In"=w127, "Waveform Task In"=w126, "Experimental Control Cluster In"=w145) -> ("error out"=w143:errorcluster, "waveform task out"=w121:refnum<k21>, "counter task out"=w125:refnum<k21>, "Experimental Control Cluster Out"=w142:T13)  [unwired: 4 in]
              n51 = call "DoExperiment.vi"("Error In"=w143, "Camera Information 2"=w139, "Acquisition Parameters"=w140, "output cluster"=w142) -> ("error out"=w124:errorcluster, "Background Image"=w137:i32[][], "Atom Image"=w136:i32[][], "output cluster 2"=w141:T13)  [unwired: 4 in]
              n52 = Increment(x=w138) -> (x+1=w134:i32)
              n53 = call <vilib>:"DAQmx Wait Until Done.vi"("task/channels in"=w125, "error in"=w124) -> ("task out"=w122:refnum<k21>, "error out"=w123:errorcluster)  [unwired: 12 in]
              n54 = call "SaveImages.vi"("Background Image"=w137, "Atoms Image"=w136, "Base Filename"=w135, "Raw Data Path"=w133, "ImageNumber"=w134) -> ("Background Image 2"=→"Background Image":i16[][], "Atoms Image 2"=→"Atom Image":i16[][])  [unwired: 9 in]
              n55 = call "WriteBatches.vi"("Variable Parameter Value"=w128, "Image Number"=w134, "String"=w135, "Raw Data Folder"=w133) -> ()  [unwired: 8 in]
            }
            n56 = local write "You Are Changing:"("A Pulseblaster Param" ("You Are Changing:")) -> ()
          }
          frame "Static Voltage" {
            n57 = Array Size(array=w157) -> (size(s)=w156:i32)
            n58 = for {
              shift-right: [w182] -> w161
              shift-left: w162 -> [w190]
              tunnel: w157 -> [w181] mode=indexing
              shift-right: [w164] -> w160
              shift-left: w159 -> [w184]
              tunnel: w158 -> [w175]
              tunnel: w156 -> [w173]
              shift-right: [w167] -> w153
              shift-left: w155 -> [w170]
              shift-right: [w166] -> w152
              shift-left: w154 -> [w169]
              i -> [w172]
              n59 = Unbundle By Name(w190) -> ("6704 Static Voltage Settings.Voltages"=w191:dbl[])
              n60 = Replace Array Subset(array=w191, new element=w181, index="Static Channel To Change") -> (w189:dbl[])
              n61 = Bundle By Name(cluster=w190, "6704 Static Voltage Settings.Voltages"=w189) -> (w188:T13)
              n62 = local read "Acquisition Parameters"() -> (w186:T4)
              n63 = local read "Camera Information"() -> (w185:T3)
              n64 = local read "Raw_Data Folder"() -> (w180:path)
              n65 = call "WriteExp.vi"("error in (no error)"=w184, "Control Task In"=w170, "Waveform Task In"=w169, "Experimental Control Cluster In"=w188) -> ("error out"=w183:errorcluster, "waveform task out"=w166:refnum<k21>, "counter task out"=w168:refnum<k21>, "Experimental Control Cluster Out"=w187:T13)  [unwired: 4 in]
              n66 = call "DoExperiment.vi"("Error In"=w183, "Camera Information 2"=w185, "Acquisition Parameters"=w186, "output cluster"=w187) -> ("error out"=w165:errorcluster, "Background Image"=w179:i32[][], "Atom Image"=w178:i32[][], "output cluster 2"=w182:T13)  [unwired: 4 in]
              n67 = Increment(x=w172) -> (x+1=w171:i32)
              n68 = call "WriteBatches.vi"("Variable Parameter Value"=w181, "Image Number"=w171, "String"=w175, "Raw Data Folder"=w180) -> ()  [unwired: 8 in]
              n69 = call "Progress Bar.vi"("Total Number"=w173, "Current Number"=w171) -> ("Scan Progress"=→"Scan Progress":dbl)  [unwired: 13 in]
              n70 = call "SaveImages.vi"("Background Image"=w179, "Atoms Image"=w178, "Base Filename"=w175, "Raw Data Path"=w180, "ImageNumber"=w171) -> ("Background Image 2"=w177:i16[][], "Atoms Image 2"=w176:i16[][])  [unwired: 9 in]
              n71 = call <vilib>:"DAQmx Wait Until Done.vi"("task/channels in"=w168, "error in"=w165) -> ("task out"=w167:refnum<k21>, "error out"=w164:errorcluster)  [unwired: 12 in]
              n72 = local write "Background Image"(w177) -> ()
              n73 = local write "Atom Image"(w176) -> ()
            }
            "You Are Changing:" <- "A Static Voltage" ("You Are Changing:")
          }
        }
        "error constant" <- w100
        n74 = local write "Start Experiment"(FALSE ("Start Experiment")) -> ()
      }
      frame "Load Experiment" {
      }
      frame "Shutdown" {
        n75 = call <userlib>:"ShutDown.vi"("error in (no error)"=w200) -> ("error out"=w196:errorcluster)  [unwired: 1 in, 1 out]
        n76 = property on="Camera Ready" class="Bool (strict)"(error in=w196, "Value"=FALSE ("Camera Ready")) -> (error out=w195:errorcluster)  [unwired: 1 in, 1 out]
        n77 = local write "Shutdown Experiment"(FALSE ("Shutdown Experiment")) -> ()
      }
    }
  }
